vi "ROI Max Bounding Box.vi"(0 "Bounding Box In 1":T1, 5 "Bounding Box In 2":T1) -> (4 "Max Bounding Box":T1)   [LabVIEW 2014]
doc: "Compares two bounding boxes and returns the box containing both"
uses:
  MSC Image_class/controls/Contour.ctl
  MSC Image_class/MSC Image.lvclass
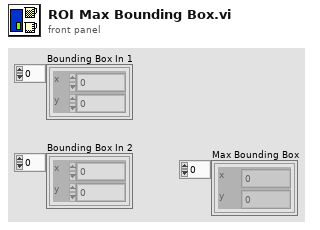
[diagram p1: front panel]
types:
  T1 = typedef "MSC Image.lvclass/Contour.ctl" = cluster{"x":i16, "y":i16}[]
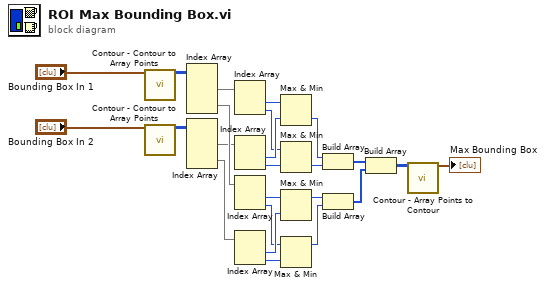
[diagram p0: block diagram]
diagram:
  n1 = call "Contour - Contour to Array Points.vi"("Contour"="Bounding Box In 1") -> ("Array Points"=w4:i16[][])  [unwired: 14 in]
  n2 = call "Contour - Contour to Array Points.vi"("Contour"="Bounding Box In 2") -> ("Array Points"=w3:i16[][])  [unwired: 14 in]
  n3 = Index Array(array=w4) -> (element #1=w18:i16[], element #2=w17:i16[])  [unwired: 4 in]
  n4 = Index Array(array=w3) -> (element #1=w15:i16[], element #2=w16:i16[])  [unwired: 4 in]
  n5 = Index Array(array=w18) -> (element #1=w14:i16, element #2=w12:i16)  [unwired: 2 in]
  n6 = Index Array(array=w15) -> (element #1=w13:i16, element #2=w11:i16)  [unwired: 2 in]
  n7 = Index Array(array=w17) -> (element #1=w10:i16, element #2=w8:i16)  [unwired: 2 in]
  n8 = Index Array(array=w16) -> (element #1=w9:i16, element #2=w7:i16)  [unwired: 2 in]
  n9 = Max & Min(x=w14, y=w13) -> (min(x,y)=w24:i16)  [unwired: 1 out]
  n10 = Max & Min(x=w12, y=w11) -> (min(x,y)=w23:i16)  [unwired: 1 out]
  n11 = Max & Min(x=w10, y=w9) -> (max(x,y)=w21:i16)  [unwired: 1 out]
  n12 = Max & Min(x=w8, y=w7) -> (max(x,y)=w22:i16)  [unwired: 1 out]
  n13 = Build Array(w24, w23) -> (w20:i16[])
  n14 = Build Array(w21, w22) -> (w19:i16[])
  n15 = Build Array(w20, w19) -> (w1:i16[][])
  n16 = call "Contour - Array Points to Contour.vi"("Array Points"=w1) -> ("Contour"=→"Max Bounding Box":T1)  [unwired: 14 in]
